vi "oa_CIC Interpolation Filter with IC.vi"(7 "reset? (True)":bool=TRUE, 8 "initial conditions":T1, 9 "CIC filter settings":T2(array[cluster]), 11 "X":dbl[](array[numeric]) format="%.2f") -> (0 "final conditions":T1, 1 "error":i32, 3 "Y":dbl[](array[numeric]) format="%.2f")   [LabVIEW 2017, in "SoundVib_Resampling.lvlib"]
uses:
  <vilib>/addons/Sound and Vibration/Order Analysis/Resample Order Tracking/SoundVib_Resampling.lvlib
  <resource>/sndvib.dll
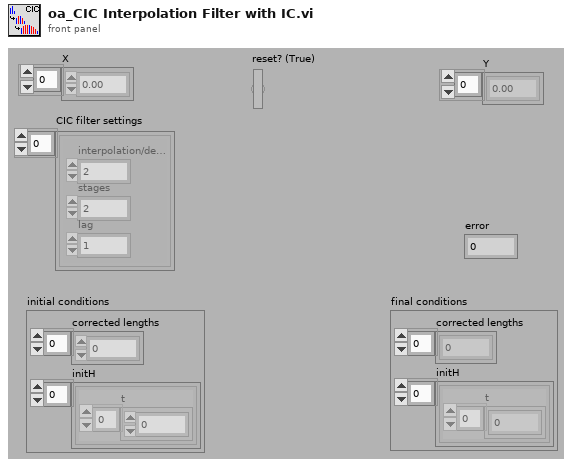
[diagram p1: front panel]
types:
  T1 = cluster{"corrected lengths":i32[], "initH":cluster{"t":dbl[]}[]}
  T2 = cluster{"interpolation/decimation factor":i32, "stages":i32, "lag":i32}[]
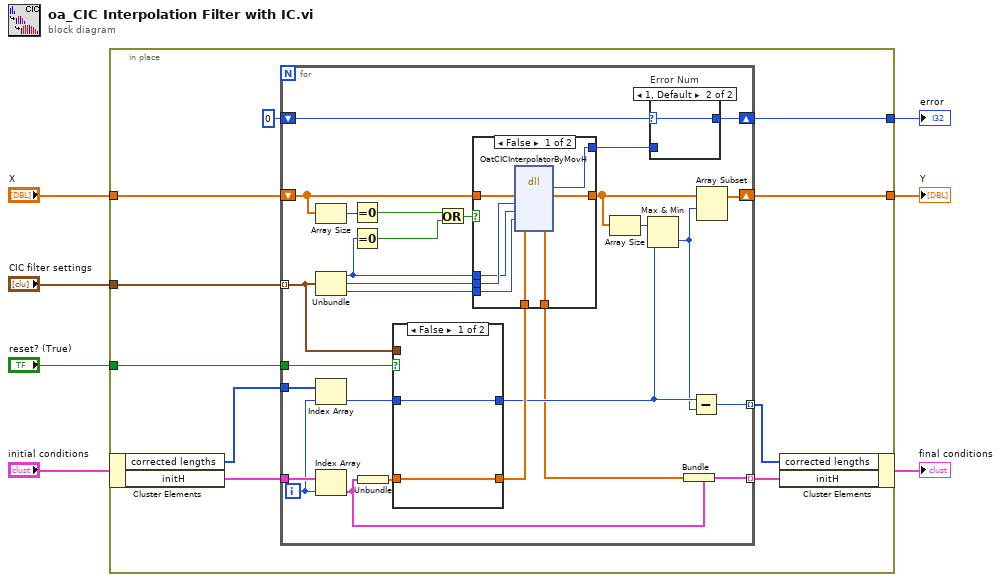
[diagram p0: block diagram]
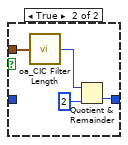
[diagram p2: hidden frame]
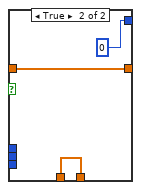
[diagram p4: hidden frame]
diagram:
  n1 = in-place {
    in-place-border: "CIC filter settings" -> [w17]
    in-place-border: "X" -> [w16]
    in-place-border: [w15] -> w5
    in-place-border: [w14] -> w4
    in-place-border: "reset? (True)" -> [w13]
    n2 = in-place-cluster #1("initial conditions") -> ("corrected lengths"=w11:i32[], "initH"=w10:cluster{"t":dbl[]}[])
    n3 = for {
      tunnel: w17 -> [w18] mode=indexing
      shift-right: [w40] -> w15
      shift-left: w16 -> [w39]
      tunnel: w10 -> [w42]
      tunnel: w13 -> [w23]
      tunnel: [w30] -> w8 mode=indexing
      tunnel: w11 -> [w29]
      shift-right: [w25] -> w14
      shift-left: 0 ("return type") -> [w26]
      tunnel: [w20] -> w9 mode=indexing
      i -> [w28]
      n4 = Array Size(array=w39) -> (size(s)=w38:i32)
      n5 = Unbundle(w18) -> ("interpolation/decimation factor"=w43:i32, "stages"=w45:i32, "lag"=w44:i32)
      n6 = Index Array(array=w29, index=w28) -> (element=w27:i32)
      n7 = Index Array(array=w42, index=w28) -> (element=w19:cluster{"t":dbl[]})
      n8 = Equal To 0?(x=w38) -> (x = 0?=w37:bool)
      n9 = Equal To 0?(x=w43) -> (x = 0?=w36:bool)
      n10 = Unbundle(w19) -> ("t"=w22:dbl[])
      n11 = case shown="False" w23 {
        tunnel: [w46 _] -> w41
        tunnel: [w47 w50] -> w32
        tunnel: w27 -> [w47 _]
        tunnel: w22 -> [w46 _]
        tunnel: w18 -> [_ w49]
        frame False {
        }
        frame True {
          n12 = call <vilib>:"oa_CIC Filter Length.vi"("CIC filter settings"=w49) -> ("CIC filter length"=w48:i32)  [unwired: 14 in]
          n13 = Quotient & Remainder(x=w48, y=2) -> (floor(x/y)=w50:i32)  [unwired: 1 out]
        }
      }
      n14 = Or(x=w37, y=w36) -> (x .or. y?=w35:bool)
      n15 = case shown="False" w35 {
        tunnel: w39 -> [w61 w64]
        tunnel: [w55 w64] -> w34
        tunnel: w45 -> [w60 _]
        tunnel: w44 -> [w59 _]
        tunnel: w43 -> [w58 _]
        tunnel: w41 -> [w57 w62]
        tunnel: [w56 w62] -> w21
        tunnel: [w54 0] -> w24
        frame False {
          n16 = dll-call lib="C:/Program Files (x86)/National Instruments/LabVIEW 2017/resource/sndvib.*" fn="OatCICInterpolatorByMovH"("xH"=w61, "stage"=w60, "dec_factor"=w58, "lag"=w59, "initH"=w57) -> ("return type"=w54:i32, "xH"=w55:dbl[], "initH"=w56:dbl[])  [unwired: 6 in, 2 out]
        }
        frame True {
        }
      }
      n17 = Array Size(array=w34) -> (size(s)=w33:i32)
      n18 = Max & Min(x=w33, y=w32) -> (min(x,y)=w31:i32)  [unwired: 1 out]
      n19 = case "Error Num" shown="1, Default" w26 {
        selector: w26 -> [_ w53]
        tunnel: [w52 w53] -> w25
        tunnel: w24 -> [w52 _]
        frame 0 {
        }
        frame 1, Default {
        }
      }
      n20 = Bundle(cluster=w19, "t"=w21) -> (w20:cluster{"t":dbl[]})
      n21 = Subtract(x=w32, y=w31) -> (x-y=w30:i32)
      n22 = Array Subset(array=w34, index=w31) -> (w40:dbl[])  [unwired: 1 in]
    }
    n23 = in-place-cluster #1("corrected lengths"=w8, "initH"=w9) -> (→"final conditions":T1)
  }
  "Y" <- w5
  "error" <- w4
